vi "Load Class.vi"(8 "error in (no error)":errorcluster, 10 "class path":path, 11 "Component Loader in":refnum<class "Component Loader.lvclass">) -> (0 "error out":errorcluster, 2 "object":refnum<class>, 3 "Component Loader out":refnum<class "Component Loader.lvclass">)   [LabVIEW 2021, in "DSF Core.lvlib" / "Component Loader.lvclass"]
uses:
  Component Loader.lvclass
  Class Not Found.vi
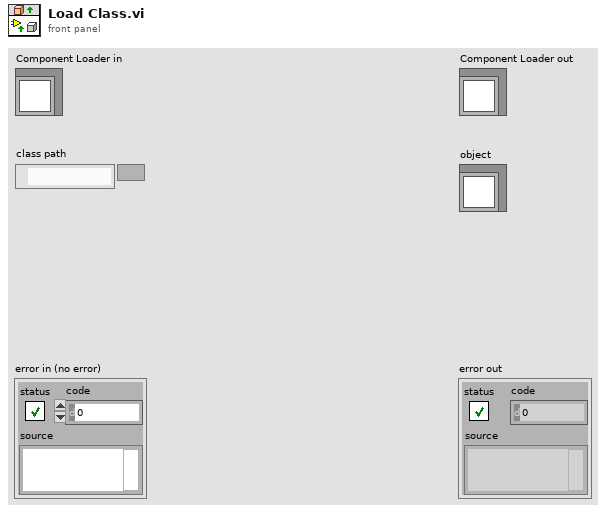
[diagram p1: front panel]
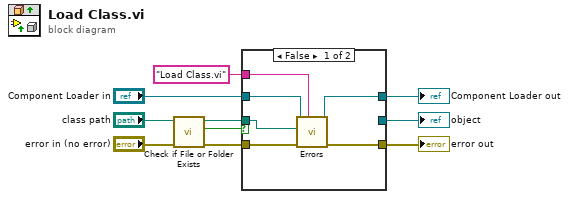
[diagram p0: block diagram]
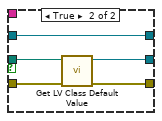
[diagram p2: hidden frame]
diagram:
  n1 = call <vilib>:"Check if File or Folder Exists.vi"("error in (no error)"="error in (no error)", "path"="class path") -> ("error out"=w9:errorcluster, "file or folder exists?"=w10:bool, "dup path"=w8:path)  [unwired: 7 in]
  n2 = case shown="False" w10 {
    tunnel: w9 -> [w16 w21]
    tunnel: w8 -> [w12 w20]
    tunnel: [_ w19] -> w5
    tunnel: [w15 w18] -> w4
    tunnel: "Component Loader in" -> [w14 w17]
    tunnel: [w13 w17] -> w2
    tunnel: "Load Class.vi" ("error source vi name") -> [w11 _]
    frame False {
      n3 = call-poly "Errors.vi"("error source vi name"=w11, "error in (no error)"=w16, "class path"=w12, "Component Loader in"=w14) -> ("error out"=w15:errorcluster, "Component Loader out"=w13:refnum<class "Component Loader.lvclass">)  [unwired: 6 in]
    }
    frame True {
      n4 = call <vilib>:"Get LV Class Default Value.vi"("error in (no error)"=w21, "class path"=w20) -> ("error out"=w18:errorcluster, "object"=w19:refnum<class>)  [unwired: 8 in]
    }
  }
  "error out" <- w4
  "Component Loader out" <- w2
  "object" <- w5
